vi "MSG display box_2.vi"(4 "2nd Button":string="Cancel", 6 "1st Button":string="OK", 7 "EN Continue":bool, 8 "error in":errorcluster, 9 "Enable":bool=TRUE, 10 "input string":string, 11 "Text.Text Colors:BG Color":u32(colorbox)=16448250) -> (0 "error out":errorcluster, 1 "Boolean":bool, 2 "Continue 2":bool)   [LabVIEW 2021]
panel:
  in  "Continue":bool
  in  "Cancel":bool
  in  "OK Button":bool
  out "String":string
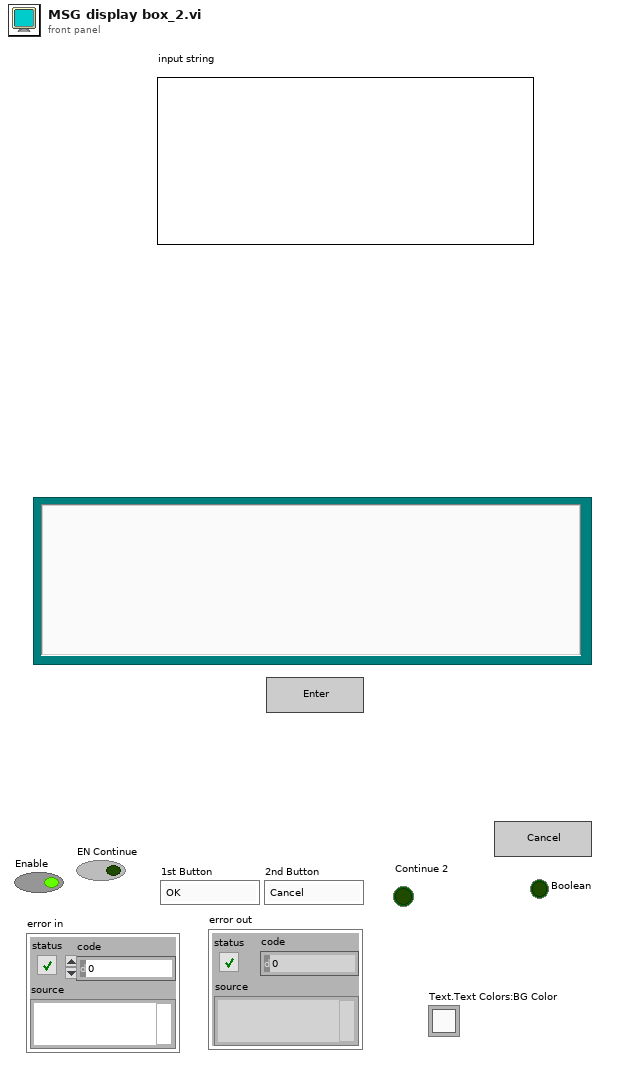
[diagram p1: front panel]
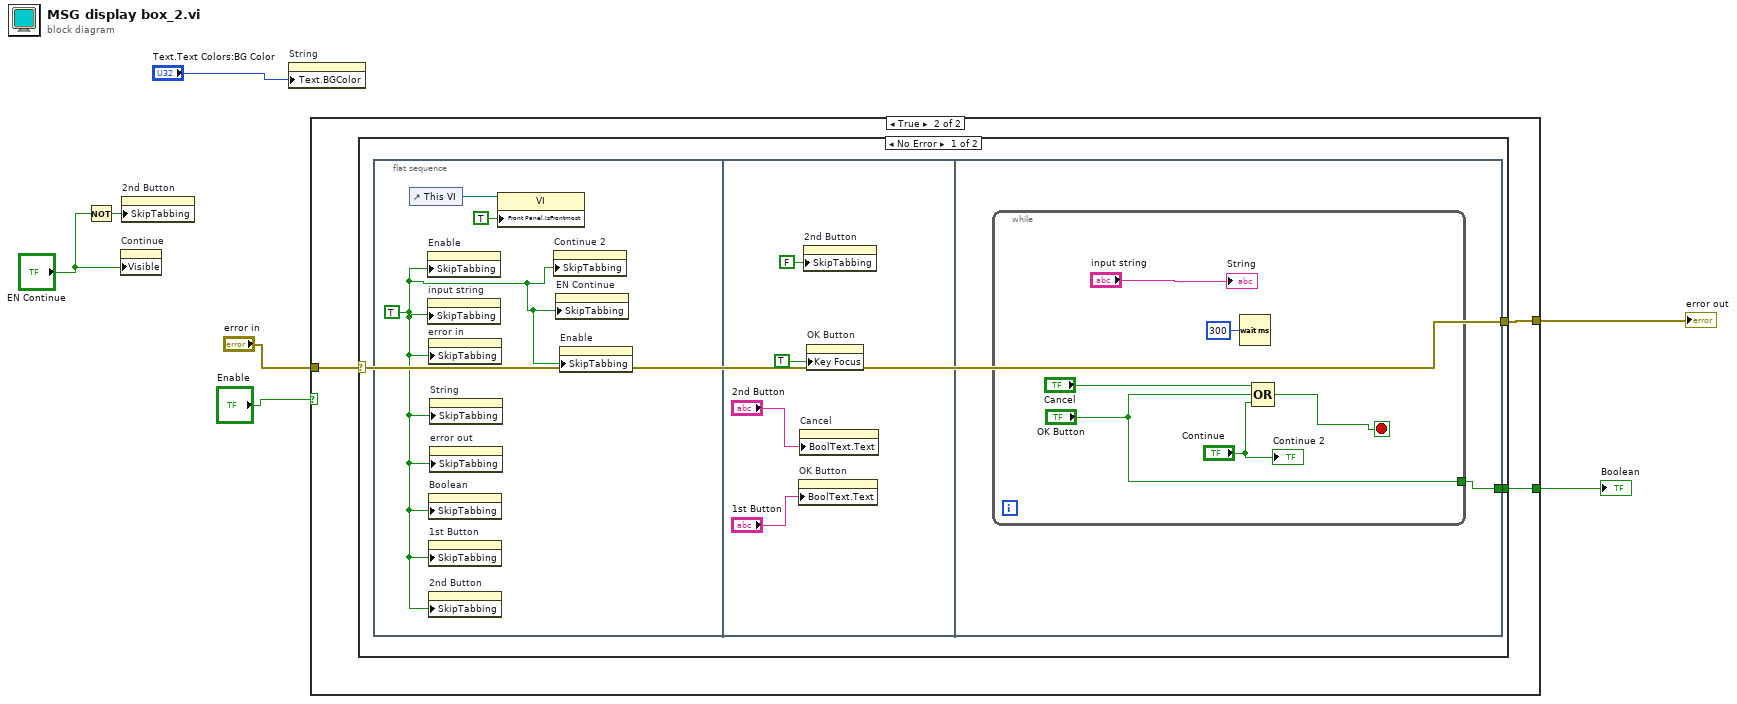
[diagram p0: block diagram]
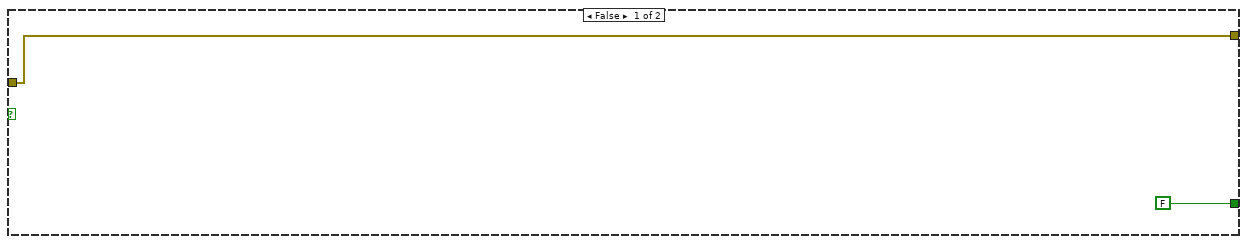
[diagram p2: hidden frame]
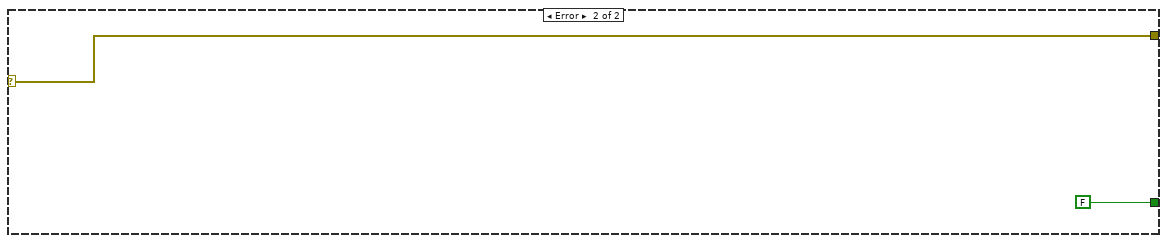
[diagram p3: hidden frame]
diagram:
  n1 = Not(x="EN Continue") -> (.not. x?=w2:bool)
  n2 = property on="Continue" class="Bool"("Visible"="EN Continue") -> ()  [unwired: 2 in, 2 out]
  n3 = property on="2nd Button" class="Str"("SkipTabbing"=w2) -> ()  [unwired: 2 in, 2 out]
  n4 = property on="String" class="Str"("Text.BGColor"="Text.Text Colors:BG Color") -> ()  [unwired: 2 in, 2 out]
  n5 = case shown="True" "Enable" {
    tunnel: "error in" -> [w9 w12]
    tunnel: [w9 w11] -> w6
    tunnel: [FALSE ("OK Button") w10] -> w4
    frame False {
    }
    frame True {
      n6 = case shown="No Error" w12 {
        selector: w12 -> [w14 w30]
        tunnel: [w14 w30] -> w11
        tunnel: [w13 FALSE ("OK Button")] -> w10
        frame No Error {
          n7 = flat-sequence {
            tunnel: [w22] -> w13
            frame #0 {
              w15 = TRUE ("Skip When Tabbing")
              n8 = control-ref of="This VI"() -> (w17:refnum<vi>)
              n9 = property on="Enable" class="Bool (strict)"("SkipTabbing"=w15) -> ()  [unwired: 2 in, 2 out]
              n10 = property on="input string" class="Str"("SkipTabbing"=w15) -> ()  [unwired: 2 in, 2 out]
              n11 = property on="error in" class="Clust (strict)"("SkipTabbing"=w15) -> ()  [unwired: 2 in, 2 out]
              n12 = property on="Boolean" class="Bool (strict)"("SkipTabbing"=w15) -> ()  [unwired: 2 in, 2 out]
              n13 = property on="1st Button" class="Str"("SkipTabbing"=w15) -> ()  [unwired: 2 in, 2 out]
              n14 = property on="2nd Button" class="Str"("SkipTabbing"=w15) -> ()  [unwired: 2 in, 2 out]
              n15 = property on="String" class="Str"("SkipTabbing"=w15) -> ()  [unwired: 2 in, 2 out]
              n16 = property on="error out" class="Clust (strict)"("SkipTabbing"=w15) -> ()  [unwired: 2 in, 2 out]
              n17 = property class="VI"(reference=w17, "Front Panel.IsFrontmost"=TRUE ("Front Panel Window:Is Frontmost")) -> ()  [unwired: 1 in, 2 out]
              n18 = property on="Continue 2" class="Bool"("SkipTabbing"=w15) -> ()  [unwired: 2 in, 2 out]
              n19 = property on="EN Continue" class="Bool (strict)"("SkipTabbing"=w15) -> ()  [unwired: 2 in, 2 out]
              n20 = property on="Enable" class="Bool (strict)"("SkipTabbing"=w15) -> ()  [unwired: 2 in, 2 out]
            }
            frame #1 {
              n21 = property on="OK Button" class="Bool"("BoolText.Text"="1st Button") -> ()  [unwired: 2 in, 2 out]
              n22 = property on="Cancel" class="Bool"("BoolText.Text"="2nd Button") -> ()  [unwired: 2 in, 2 out]
              n23 = property on="2nd Button" class="Str"("SkipTabbing"=FALSE ("Skip When Tabbing")) -> ()  [unwired: 2 in, 2 out]
              n24 = property on="OK Button" class="Bool"("Key Focus"=TRUE) -> ()  [unwired: 2 in, 2 out]
            }
            frame #2 {
              n25 = while {
                tunnel: ["OK Button"] -> w22
                stop <- w23 stop-if-true
                n26 = Wait (ms)(milliseconds to wait=u32 300) -> ()  [unwired: 1 out]
                n27 = Compound Arithmetic op=OR("Cancel", "OK Button", "Continue") -> (w23:bool)
                "String" <- "input string"
                "Continue 2" <- "Continue"
              }
            }
          }
        }
        frame Error {
        }
      }
    }
  }
  "error out" <- w6
  "Boolean" <- w4
